vi "Search Filter 1D Array of String.vi"(5 "Ignore case? (F)":bool, 7 "Method (Contains Search String)":T1(ring), 10 "Search String":string, 11 "String Array to Search":string[](array[string])) -> (1 "Filtered Array":string[](array[string]), 2 "Indicies Found":i32[](array[numeric]), 3 "Matching Elements":string[](array[string]))   [LabVIEW 2017, in "Front Panel Publisher.lvlib"]
doc: "This VI will search and filter a 1D array of string passed into <b>String Array to Search</b>. This array will be searched using the method defined in <b>Method</b> using the string <b>Search String</b> as the criteria for the search. The output of <b>Filtered Array</b> will contain the input <B>String Array to Search</B>, with the elements deleted that matched the search settings. The output of <B>Matching Elements</B> will be all of the elements from <B>String Array to Search</B> that met the search settings.\n\nThis VI can search for a the elements that contain the search string, start with the search string, or end with the search string.\n\nAdditionally the <b>Indicies Found</b> will contain the places where the search criteria were found.\n\nThe search can also be modified to <b>Ignore case</b> which will cause the search string to ignore capitialization."
uses:
  Front Panel Publisher.lvlib
  <userlib>/_OpenG.lib/array/array.llb/Delete Elements from 1D Array (String)__ogtk.vi
  <userlib>/_OpenG.lib/array/array.llb/Search 1D Array (Boolean)__ogtk.vi
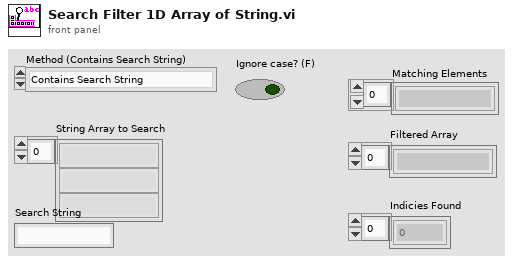
[diagram p1: front panel]
types:
  T1 = enum16{"Contains Search String", "Starts With Search String", "Ends With Search String", "Exact String"}
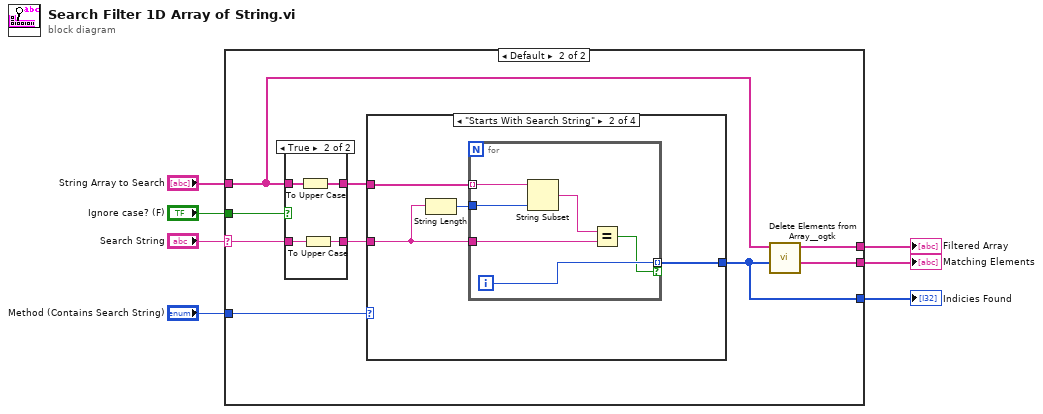
[diagram p0: block diagram]
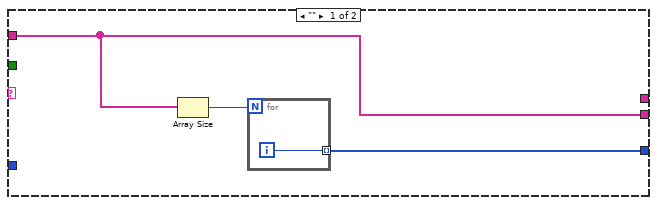
[diagram p2: hidden frame]
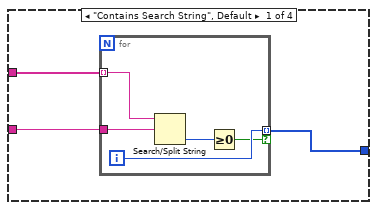
[diagram p4: hidden frame]
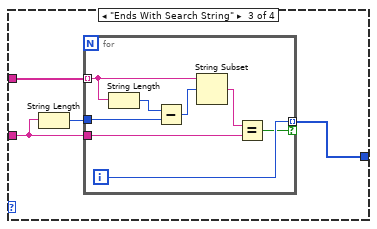
[diagram p5: hidden frame]
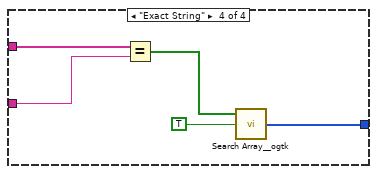
[diagram p6: hidden frame]
diagram:
  n1 = case shown="Default" "Search String" {
    selector: "Search String" -> [_ w12]
    tunnel: "Method (Contains Search String)" -> [_ w20]
    tunnel: "Ignore case? (F)" -> [_ w19]
    tunnel: [w9 w16] -> w5
    tunnel: "String Array to Search" -> [w8 w15]
    tunnel: [_ w14] -> w3
    tunnel: [w8 w13] -> w2
    frame "" {
      n2 = Array Size(array=w8) -> (size(s)=w10:i32)
      n3 = for {
        N: w10 -> [_]
        tunnel: [w11] -> w9 mode=indexing
        i -> [w11]
      }
    }
    frame Default {
      n4 = case shown="True" w19 {
        tunnel: w12 -> [w21 w24]
        tunnel: w15 -> [w22 w26]
        tunnel: [w22 w25] -> w18
        tunnel: [w21 w23] -> w17
        frame False {
        }
        frame True {
          n5 = To Upper Case(1:w26) -> (0:w25:string[])
          n6 = To Upper Case(1:w24) -> (0:w23:string)
        }
      }
      n7 = case shown="\"Starts With Search String\"" w20 {
        tunnel: w17 -> [w29 w36 w47 w60]
        tunnel: w18 -> [w28 w38 w48 w61]
        tunnel: [w27 w35 w45 w57] -> w16
        frame "Contains Search String", Default {
          n8 = for {
            tunnel: w28 -> [w34] mode=indexing
            tunnel: w29 -> [w33]
            tunnel: [w32] -> w27 mode=indexing if=w30
            i -> [w32]
            n9 = Search/Split String(string=w34, search string/char (-)=w33) -> (offset of match=w31:i32)  [unwired: 1 in, 2 out]
            n10 = Greater Or Equal To 0?(x=w31) -> (x >= 0?=w30:bool)
          }
        }
        frame "Starts With Search String" {
          n11 = String Length(string=w36) -> (length=w37:i32)
          n12 = for {
            tunnel: w38 -> [w43] mode=indexing
            tunnel: w37 -> [w44]
            tunnel: w36 -> [w41]
            tunnel: [w40] -> w35 mode=indexing if=w39
            i -> [w40]
            n13 = String Subset(string=w43, length (rest)=w44) -> (substring=w42:string)  [unwired: 1 in]
            n14 = Equal?(x=w42, y=w41) -> (x = y?=w39:bool)
          }
        }
        frame "Ends With Search String" {
          n15 = String Length(string=w47) -> (length=w46:i32)
          n16 = for {
            tunnel: w48 -> [w54] mode=indexing
            tunnel: w47 -> [w55]
            tunnel: w46 -> [w52]
            tunnel: [w50] -> w45 mode=indexing if=w49
            i -> [w50]
            n17 = String Length(string=w54) -> (length=w53:i32)
            n18 = Subtract(x=w53, y=w52) -> (x-y=w51:i32)
            n19 = String Subset(string=w54, offset (0)=w51) -> (substring=w56:string)  [unwired: 1 in]
            n20 = Equal?(x=w56, y=w55) -> (x = y?=w49:bool)
          }
        }
        frame "Exact String" {
          n21 = Equal?(x=w61, y=w60) -> (x = y?=w59:bool[])
          n22 = call-poly <userlib>:"Search Array__ogtk.vi"("Array"=w59, "Element Data"=TRUE) -> ("Indices of Elements"=w57:i32[])  [unwired: 7 in]
        }
      }
      n23 = call-poly <userlib>:"Delete Elements from Array__ogtk.vi"("indices"=w16, "array"=w15) -> ("deleted elements"=w13:string[], "array w/ subset deleted"=w14:string[])  [unwired: 8 in]
    }
  }
  "Filtered Array" <- w3
  "Indicies Found" <- w5
  "Matching Elements" <- w2
